vi "Read CtlRef.vi"(8 "error in (no error)":errorcluster, 11 "ControlMouseDownMsg in":refnum<class "ControlMouseDownMsg.lvclass">) -> (0 "error out":errorcluster, 2 "CtlRef":refnum<vi>, 3 "ControlMouseDownMsg out":refnum<class "ControlMouseDownMsg.lvclass">)   [LabVIEW 2018, in "MVA Framework.lvlib" / "ActorEvents.lvlib" / "ControlMouseDownMsg.lvclass"]
uses:
  ControlMouseDownMsg.lvclass
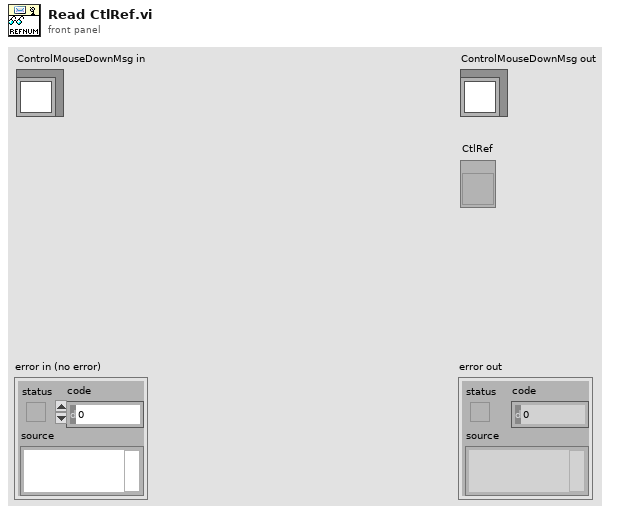
[diagram p1: front panel]
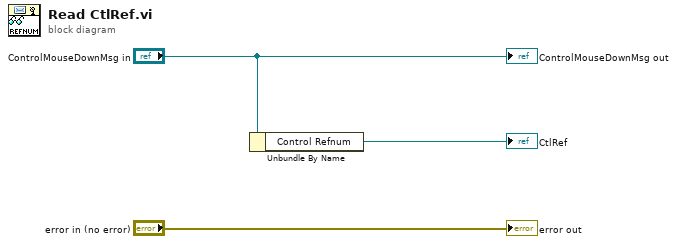
[diagram p0: block diagram]
diagram:
  n1 = Unbundle By Name("ControlMouseDownMsg in") -> ("Control Refnum"=→"CtlRef":refnum<vi>)
  "error out" <- "error in (no error)"
  "ControlMouseDownMsg out" <- "ControlMouseDownMsg in"
